vi "19572_read_UT_status.vi"(8 "error in (no error)":errorcluster, 10 "timeout":dbl=10.0 format="%0.2f", 11 "task/channles in":refnum<k21>) -> (0 "error out":errorcluster, 1 "Under Test":bool, 3 "task out":refnum<k21>)   [LabVIEW 2015]
uses:
  <vilib>/DAQmx/read.llb/DAQmx Read (Digital 1D Bool 1Chan 1Samp).vi
  <vilib>/DAQmx/miscellaneous.llb/DAQmx Fill In Error Info.vi
panel:
  # "Read CHROMA 19572 UNDER TEST LED status"
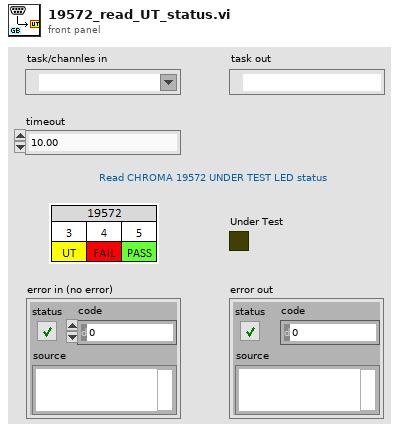
[diagram p1: front panel]
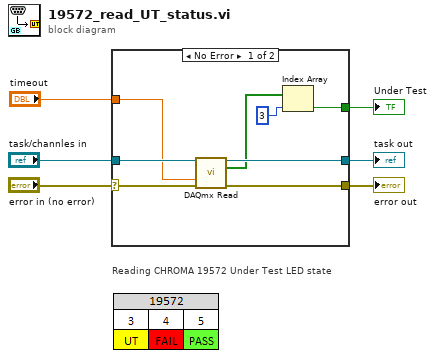
[diagram p0: block diagram]
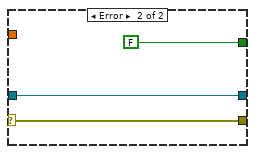
[diagram p2: hidden frame]
diagram:
  # "Reading CHROMA 19572 Under Test LED state"
  n1 = case shown="No Error" "error in (no error)" {
    selector: "error in (no error)" -> [w8 w15]
    tunnel: [w14 w15] -> w6
    tunnel: [w13 FALSE ("Boolean")] -> w5
    tunnel: "task/channles in" -> [w12 w16]
    tunnel: [w10 w16] -> w3
    tunnel: "timeout" -> [w7 _]
    frame No Error {
      n2 = call-poly <vilib>:"DAQmx Read.vi"("task/channels in"=w12, "timeout"=w7, "error in"=w8) -> ("task out"=w10:refnum<k21>, "data"=w9:bool[], "error out"=w14:errorcluster)  [unwired: 10 in]
      n3 = Index Array(array=w9, index=3) -> (element=w13:bool)
    }
    frame Error {
    }
  }
  "error out" <- w6
  "Under Test" <- w5
  "task out" <- w3
